vi "FC_Parse_Team_Info.vi"(8 "Error In":errorcluster, 10 "All Team Data":string) -> (0 "Error Out":errorcluster, 2 "Team Data Cluster":T1)   [LabVIEW 2014, in "FC_FIRST Client.lvlib"]
doc: "This VI parses the data of a team and returns a cluster of the team attributes"
uses:
  FC_FIRST Client.lvlib
  FC_Team Attributes.ctl
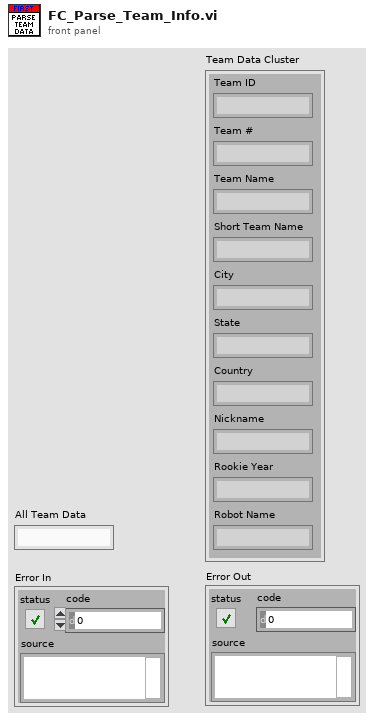
[diagram p1: front panel]
types:
  T1 = typedef "FC_FIRST Client.lvlib/FC_Team Attributes.ctl" = cluster{"Team ID":string, "Team #":string, "Team Name":string, "Short Team Name":string, "City":string, "State":string, "Country":string, "Nickname":string, "Rookie Year":string, "Robot Name":string}
  T2 = cluster{"[0]":string, "[1]":string, "[2]":string, "[3]":string, "[4]":string, "[5]":string, "[6]":string, "[7]":string, "[8]":string, "[9]":string}
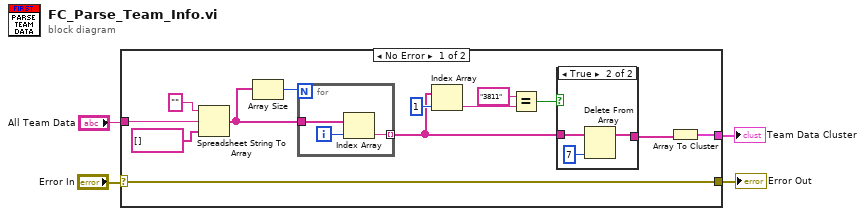
[diagram p0: block diagram]
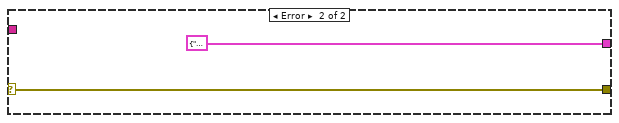
[diagram p3: hidden frame]
diagram:
  n1 = case shown="No Error" "Error In" {
    selector: "Error In" -> [w14 w26]
    tunnel: "All Team Data" -> [w15 _]
    tunnel: [w14 w26] -> w2
    tunnel: [w13 T2 {"[0]"="", "[1]"="", "[2]"="", "[3]"="", "[4]"="", "[5]"="", "[6]"="", "[7]"="", "[8]"="", "[9]"=""}] -> w1
    frame No Error {
      n2 = Spreadsheet String To Array(format string="", spreadsheet string=w15, array type (2D Dbl)=string[] []) -> (array=w11:string[])  [unwired: 1 in]
      n3 = Array Size(array=w11) -> (size(s)=w12:i32)
      n4 = for {
        N: w12 -> [_]
        tunnel: [w24] -> w7 mode=indexing
        tunnel: w11 -> [w23]
        i -> [w22]
        n5 = Index Array(array=w23, index=w22) -> (element=w24:string)
      }
      n6 = Index Array(array=w7, index=1) -> (element=w9:string)
      n7 = Equal?(x="3811", y=w9) -> (x = y?=w5:bool)
      n8 = case shown="True" w5 {
        tunnel: [w18 w19] -> w6
        tunnel: w7 -> [w18 w21]
        frame False {
        }
        frame True {
          n9 = Delete From Array(array=w21, index=7) -> (array with subset deleted=w19:string[])  [unwired: 1 in, 1 out]
        }
      }
      n10 = Array To Cluster(array=w6) -> (cluster=w13:T2)
    }
    frame Error {
    }
  }
  "Error Out" <- w2
  "Team Data Cluster" <- w1
